vi "setStyleStrategy.vi"(8 "Error In":errorcluster, 10 "s":T1=1 items=["PreferDefault"=1, "PreferBitmap"=2, "PreferDevice"=4, "PreferOutline"=8, "ForceOutline"=16, "PreferMatch"=32, "PreferQuality"=64, "PreferAntialias"=128, "NoAntialias"=256, "OpenGLCompatible"=512, "ForceIntegerMetrics"=1024, "NoSubpixelAntialias"=2048, "NoFontMerging"=32768], 11 "QFont In":refnum<class "QFont.lvclass">) -> (0 "Error Out":errorcluster, 3 "QFont Out":refnum<class "QFont.lvclass">)   [LabVIEW 2014, in "QFont.lvclass"]
doc: "LabVIEW-specific documentation is not yet available. See <b>http://doc.qt.io/qt-5/QFont.html#setStyleStrategy</b>"
uses:
  QFont.lvclass
  StyleStrategy.ctl
  LQ Core/LQSerialData/LQSerialData.lvclass/LQSerialData.ctl
  LQ Core/LQ Core.lvlib
  LQ Core/LQSerialData/LQSerialData.lvclass
panel:
  # "Copyright (c) 2016 Sze Howe Koh\n\nThis Source Code Form is subject to the terms of the Mozilla Public\nLicense, v. 2.0. If a copy of the MPL was not distributed with this\nfile, You can obtain one at http://mozilla.org/MPL/2.0/."
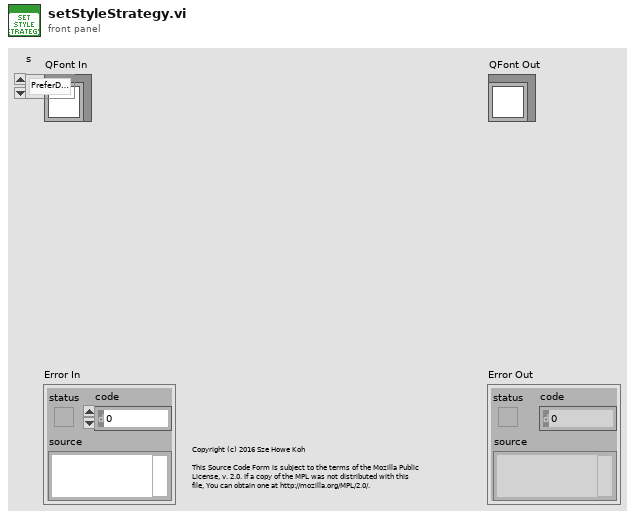
[diagram p1: front panel]
types:
  T1 = typedef "QFont.lvclass/StyleStrategy.ctl" = i32
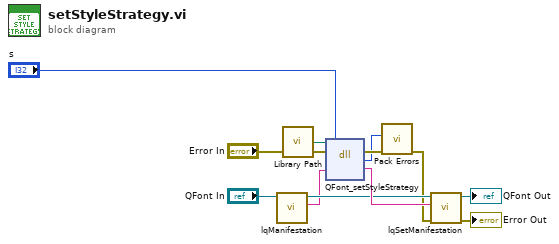
[diagram p0: block diagram]
diagram:
  n1 = call "lqManifestation.vi"("LQSerialData in"="QFont In") -> ("Manifestation"=w7:string, "LQSerialData out"=w8:refnum<class "QFont.lvclass">)  [unwired: 9 in]
  n2 = call "Library Path.vi"() -> ("Library Path"=w6:path)
  n3 = dll-call lib="?" fn="QFont_setStyleStrategy"(path in=w6, error in="Error In", "_instance"=w7, "s"="s") -> (error out=w5:errorcluster, w4:i32, "_instance"=w10:string)  [unwired: 2 in, 1 out]
  n4 = call "Pack Errors.vi"("Error In"=w5, "Error Code"=w4) -> ("Error Out"=w3:errorcluster)  [unwired: 9 in]
  n5 = call "lqSetManifestation.vi"("Error In"=w3, "Manifestation"=w10, "LQSerialData in"=w8) -> ("Error Out"=→"Error Out":errorcluster, "LQSerialData out"=→"QFont Out":refnum<class "QFont.lvclass">)  [unwired: 7 in]
